vi "Array Average.vi"() -> ()   [LabVIEW 2019]
panel:
  out "Average":dbl
  in  "Array":dbl[](array[numeric])
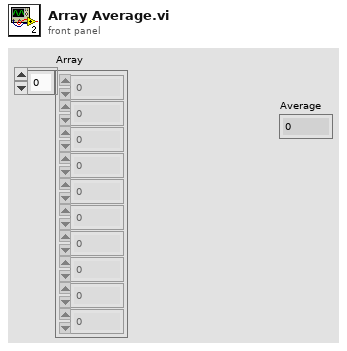
[diagram p1: front panel]
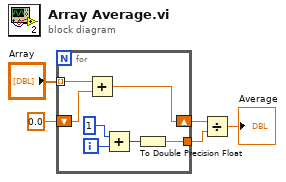
[diagram p0: block diagram]
diagram:
  n1 = for {
    shift-right: [w11] -> w3
    shift-left: 0.0 -> [w12]
    tunnel: "Array" -> [w10] mode=indexing
    tunnel: [w6] -> w2
    i -> [w8]
    n2 = Add(x=w10, y=w12) -> (x+y=w11:dbl)
    n3 = Add(x=1, y=w8) -> (x+y=w7:i32)
    n4 = To Double Precision Float(number=w7) -> (double precision float=w6:dbl)
  }
  n5 = Divide(x=w3, y=w2) -> (x/y=→"Average":dbl)
